vi "Apply Display State to Front Panel and Signal Configuration.vi"(7 "Data In":T1, 10 "references":T2, 11 "Display State In":T3) -> (3 "Display State Out":T3, 5 "Data Out":T1)   [LabVIEW 2017, in "Test Signal Configuration.xctl"]
uses:
  <vilib>/addons/_XControls/Function Generator Configuration/Test Signal Configuration.xctl
  <vilib>/addons/_XControls/Function Generator Configuration/Controls/State.ctl
  <vilib>/addons/_XControls/Function Generator Configuration/Controls/references.ctl
  <vilib>/addons/_XControls/Function Generator Configuration/Controls/Data.ctl
  <vilib>/addons/_NISVFA/_Generation/Signal Generation/SV Signal/SV Signal.lvclass
  <vilib>/addons/_NISVFA/_Generation/Signal Generation/SV Signal/sv_System Timing Model.ctl
  <vilib>/addons/_NISVFA/_Generation/Signal Generation/SV Sinusoid/SV Sinusoid.lvclass
  C:/Program Files (x86)/National Instruments/LabVIEW 2017/vi.lib/addons/_NISVFA/_Generation/Signal Generation/SV Signal/SV Signal.lvclass
  <vilib>/addons/_NISVFA/_Generation/Signal Generation/SV Multitone/SV Multitone.lvclass
  <vilib>/addons/_NISVFA/_Generation/Signal Generation/SV Discrete Sweep/SV Discrete Sweep.lvclass
  C:/Program Files (x86)/National Instruments/LabVIEW 2017/vi.lib/addons/_NISVFA/_Generation/Signal Generation/SV Function/SV Function.lvclass
  <vilib>/addons/_NISVFA/_Generation/Signal Generation/SV Continuous Sweep/SV Continuous Sweep.lvclass
  <vilib>/addons/_NISVFA/_Generation/Signal Generation/SV Noise/SV Noise.lvclass
  <vilib>/addons/_NISVFA/_Generation/Signal Generation/SV Signal/Write Sample Rate.vi
  <vilib>/addons/_NISVFA/_Generation/Signal Generation/SV Signal/Write Minimum Value.vi
  <vilib>/addons/_NISVFA/_Generation/Signal Generation/SV Signal/Write Maximum Value.vi
  <vilib>/addons/_NISVFA/_Generation/Signal Generation/SV Signal/Write DC Offset.vi
  <vilib>/addons/_NISVFA/_Generation/Signal Generation/SV Signal/Write System Timing Model.vi
  <vilib>/addons/_NISVFA/_Generation/Signal Generation/SV Noise/Configure Pink Noise.vi
  <vilib>/addons/_NISVFA/_Generation/Signal Generation/SV Noise/Configure White Noise.vi
  <vilib>/addons/_NISVFA/_Generation/Signal Generation/SV Continuous Sweep/Configure Continuous Sweep.vi
  <vilib>/addons/_NISVFA/_Generation/Signal Generation/SV Signal/Write Measurement Duration.vi
  <vilib>/addons/_NISVFA/_Generation/Signal Generation/SV Function/Write Measurement Cycles.vi
  <vilib>/addons/_NISVFA/_Generation/Signal Generation/SV Discrete Sweep/Configure Frequency Sweep at Constant Amplitude.vi
  <vilib>/addons/_NISVFA/_Generation/Signal Generation/SV Multitone/Configure Multitone (Custom).vi
  <vilib>/addons/_NISVFA/_Generation/Signal Generation/SV Sinusoid/Configure Sine.vi
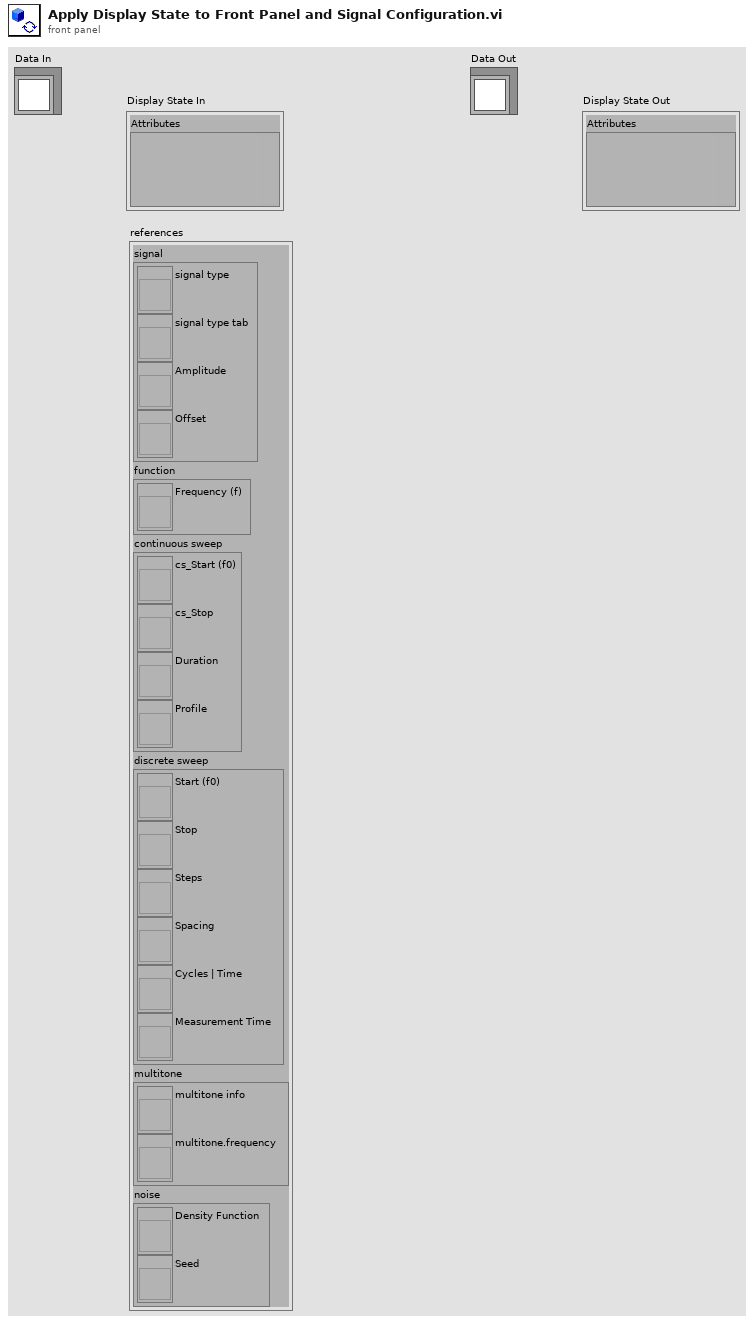
[diagram p1: front panel]
types:
  T1 = typedef "Test Signal Configuration.xctl/Data.ctl" = refnum<class "SV Signal.lvclass">
  T2 = typedef "Test Signal Configuration.xctl/references.ctl" = cluster{"signal":cluster{"signal type":refnum<vi>, "signal type tab":refnum<vi>, "Amplitude":refnum<vi>, "Offset":refnum<vi>}, "function":cluster{"Frequency (f)":refnum<vi>}, "continuous sweep":cluster{"cs_Start (f0)":refnum<vi>, "cs_Stop":refnum<vi>, "Duration":refnum<vi>, "Profile":refnum<vi>}, "discrete sweep":cluster{"Start (f0)":refnum<vi>, "Stop":refnum<vi>, "Steps":refnum<vi>, "Spacing":refnum<vi>, "Cycles | Time":refnum<vi>, "Measurement Time":refnum<vi>}, "multitone":cluster{"multitone info":refnum<vi>, "multitone.frequency":refnum<vi>}, "noise":cluster{"Density Function":refnum<vi>, "Seed":refnum<vi>}}
  T3 = typedef "Test Signal Configuration.xctl/State.ctl" = cluster{"Attributes":variant}
  T4 = typedef "SV Signal.lvclass/sv_System Timing Model.ctl" = i64
  T5 = typedef "Test Signal Configuration.xctl/signal type.ctl" = enum32{"None", "Tone", "Multitone", "Discrete Sweep", "Continuous Sweep", "Noise"}
  T6 = cluster{"Signal":cluster{"Sample Rate":cluster{"name":string, "default":dbl}, "Signal Type":cluster{"name":string, "signal type":T5}, "Amplitude":cluster{"name":string, "default":dbl}, "Offset":cluster{"name":string, "default":dbl}}, "Function":cluster{"Info":cluster{"name":string, "default":variant}, "Type":cluster{"name":string, "default":u16}, "Frequency":cluster{"name":string, "default":dbl}, "Phase":cluster{"name":string, "default":dbl}}, "Continuous Sweep":cluster{"Info":cluster{"name":string, "default":variant}, "Start":cluster{"name":string, "default":dbl}, "Stop":cluster{"name":string, "default":dbl}, "Duration":cluster{"name":string, "default":dbl}, "Profile":cluster{"name":string, "default":enum16{"Linear", "Logarithmic"}}}, "Discrete Sweep":cluster{"Info":cluster{"name":string, "default":variant}, "Start":cluster{"name":string, "default":dbl}, "Stop":cluster{"name":string, "default":dbl}, "Cycles":cluster{"name":string, "default":dbl}, "Time":cluster{"name":string, "default":dbl}, "Spacing":cluster{"name":string, "default":enum16{"Linear", "Logarithmic"}}, "Steps":cluster{"name":string, "default":i32}}, "Multitone":cluster{"Info":cluster{"name":string, "multitone info":cluster{"frequency":dbl, "amplitude":dbl, "phase":dbl}[]}}, "Noise":cluster{"Info":cluster{"name":string, "default":variant}, "Type":cluster{"name":string, "default":u16}, "Amplitude PDF":cluster{"name":string, "default":enum16{"Gaussian", "Rectangular", "Triangular"}}, "Level":cluster{"name":string, "default":dbl}, "Seed":cluster{"name":string, "default":i32}}, "Configuration":cluster{"Min Frequency":cluster{"name":string, "default":dbl}, "Max Frequency":cluster{"name":string, "default":dbl}, "Max Amplitude":cluster{"name":string, "default":dbl}}}
  T7 = enum8{"Enabled", "Disabled", "Disabled and Grayed Out"}
  T8 = cluster{"frequency":dbl, "amplitude":dbl, "phase":dbl}[]
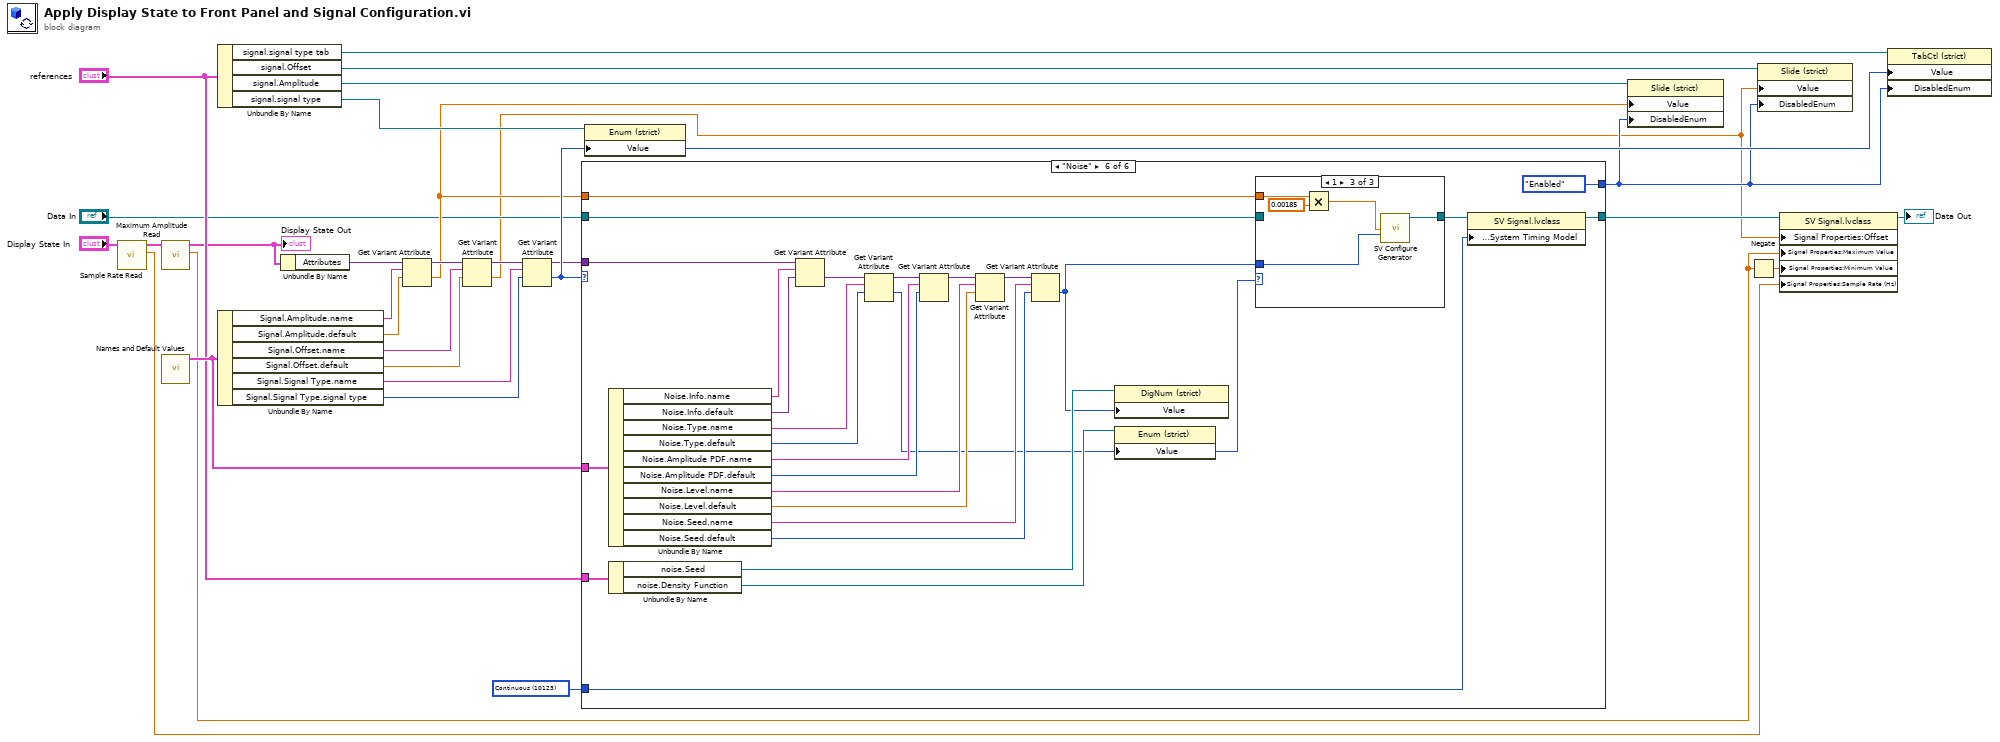
[diagram p0: block diagram]
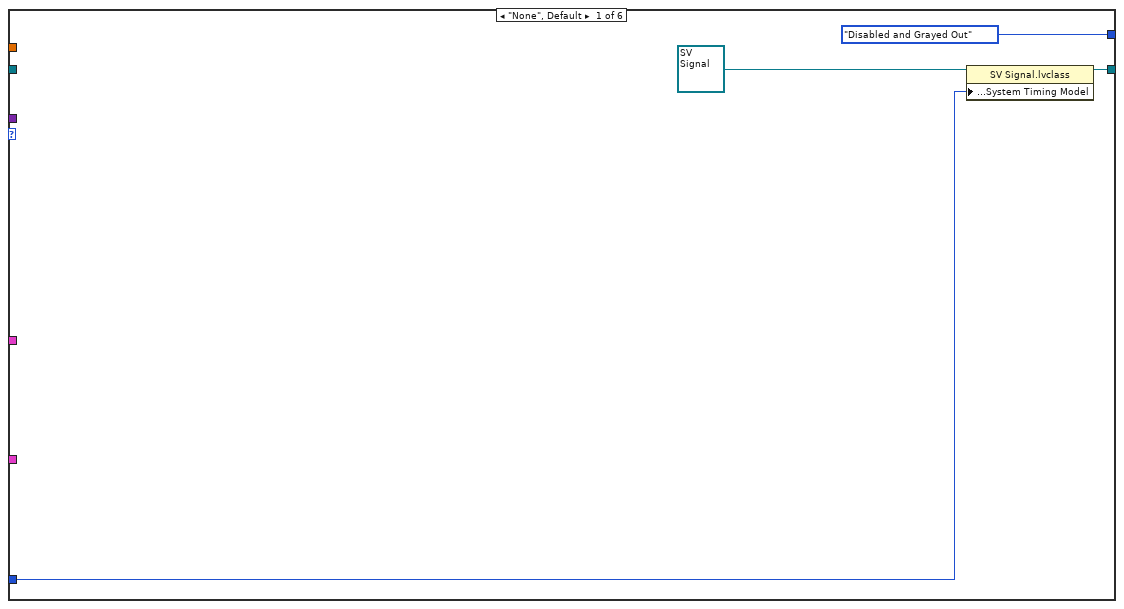
[diagram p2: hidden frame]
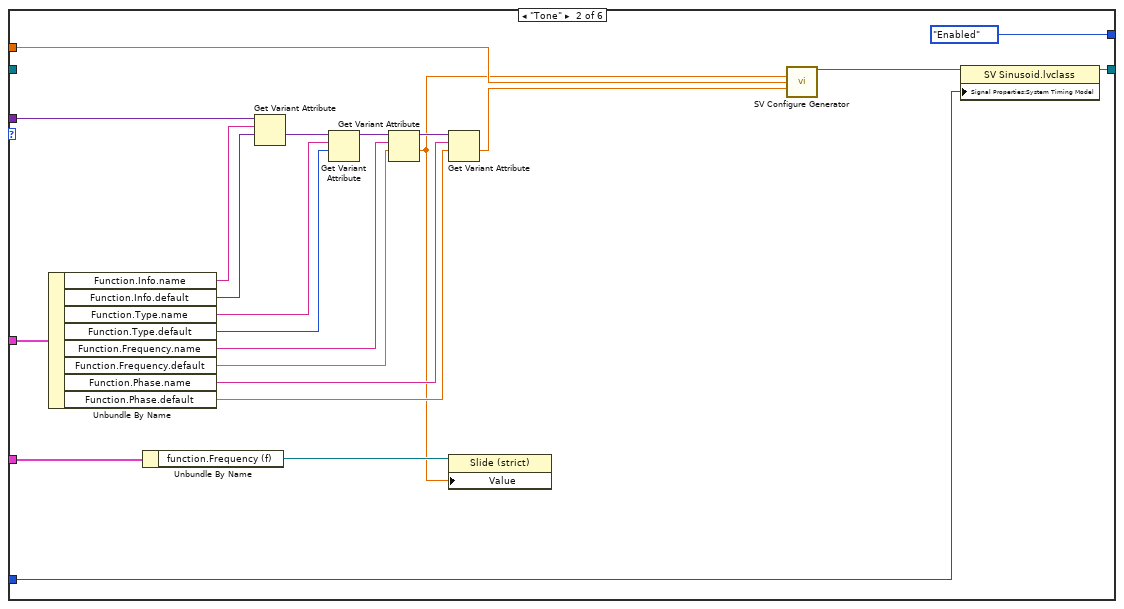
[diagram p3: hidden frame]
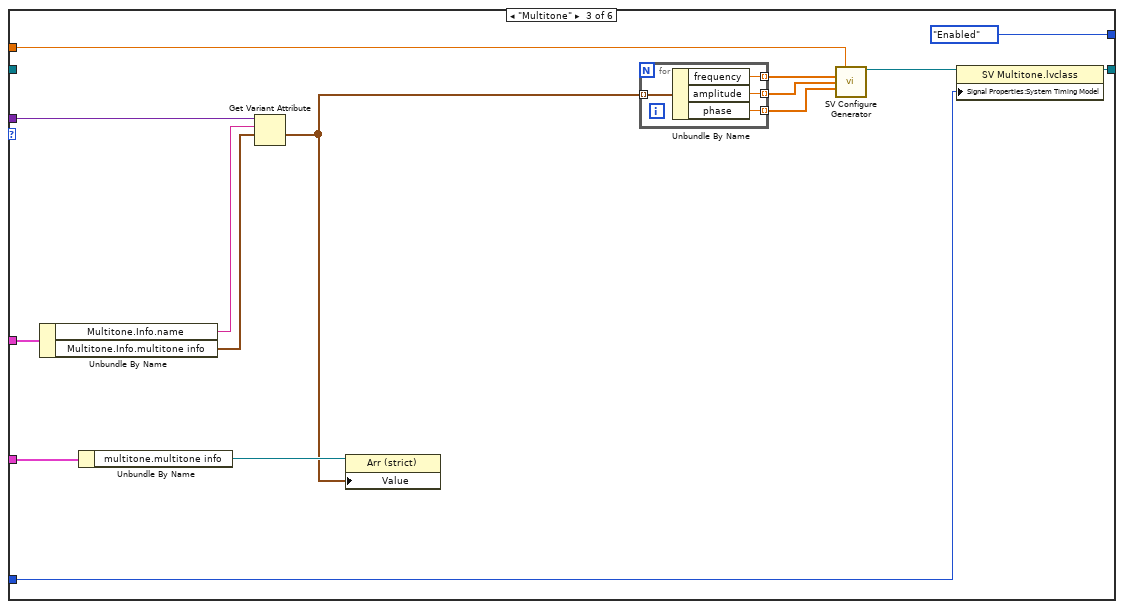
[diagram p4: hidden frame]
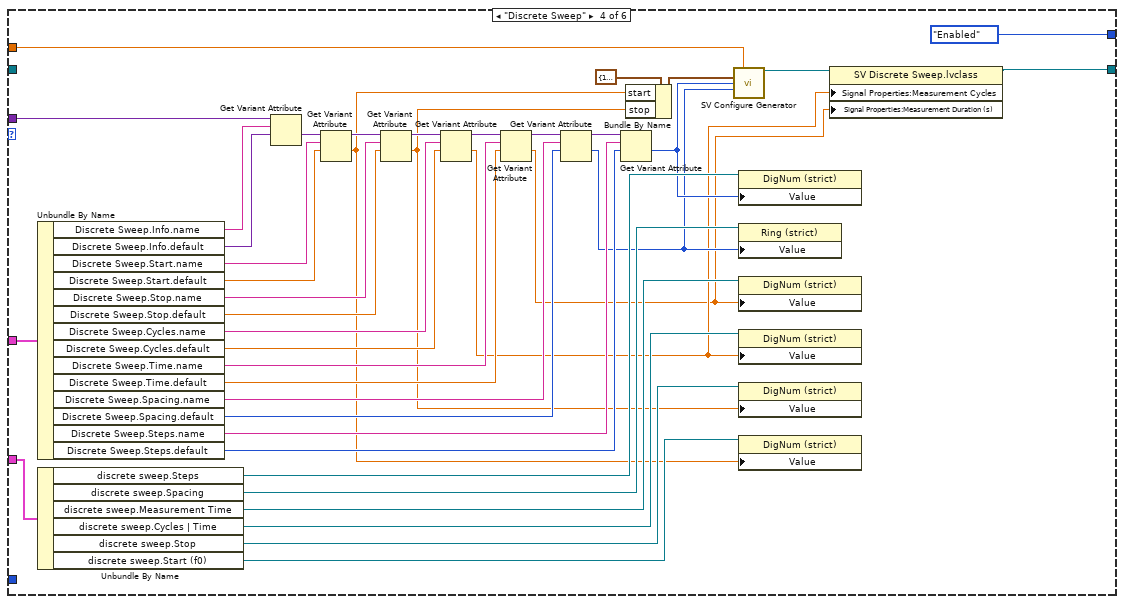
[diagram p5: hidden frame]
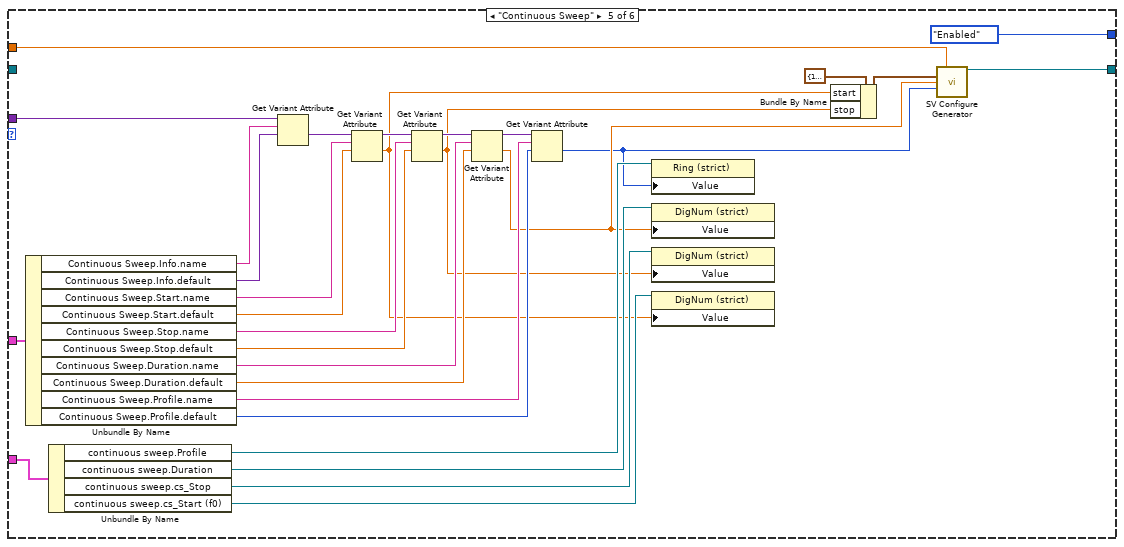
[diagram p6: hidden frame]
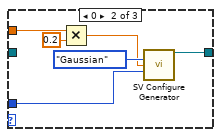
[diagram p8: hidden frame]
diagram:
  w8 = T4 10123 items=["Finite"=10178, "-"=-1, "Continuous"=10123, "-"=-2, "Settled"=110123, "Averaged"=210123, "Discrete Sweep"=310123, "Continuous Sweep"=410123] ("System Timing Model")
  n1 = call <vilib>:"Sample Rate Read.vi"("Display State In"="Display State In") -> ("Value"=w4:dbl, "Display State Out"=w5:T3)  [unwired: 4 in, 1 out]
  n2 = call <vilib>:"Maximum Amplitude Read.vi"("Display State In"=w5) -> ("Value"=w1:dbl, "Display State Out"=w7:T3)  [unwired: 4 in, 1 out]
  "Display State Out" <- w7
  n3 = call <vilib>:"Names and Default Values.vi"() -> ("Names and Default Values"=w14:T6)  [unwired: 11 in]
  n4 = Unbundle By Name("references") -> ("signal.signal type tab"=w25:refnum<vi>, "signal.Offset"=w24:refnum<vi>, "signal.Amplitude"=w23:refnum<vi>, "signal.signal type"=w16:refnum<vi>)
  n5 = Unbundle By Name(w14) -> ("Signal.Amplitude.name"=w30:string, "Signal.Amplitude.default"=w29:dbl, "Signal.Offset.name"=w27:string, "Signal.Offset.default"=w26:dbl, "Signal.Signal Type.name"=w20:string, "Signal.Signal Type.signal type"=w19:T5)
  n6 = Unbundle By Name(w7) -> ("Attributes"=w21:variant)
  n7 = Get Variant Attribute(Variant=w21, name=w30, default value (empty Variant)=w29) -> (duplicate Variant=w28:variant, value=w12:dbl)  [unwired: 1 in, 2 out]
  n8 = Get Variant Attribute(Variant=w28, name=w27, default value (empty Variant)=w26) -> (duplicate Variant=w18:variant, value=w3:dbl)  [unwired: 1 in, 2 out]
  n9 = Get Variant Attribute(Variant=w18, name=w20, default value (empty Variant)=w19) -> (duplicate Variant=w17:variant, value=w22:T5)  [unwired: 1 in, 2 out]
  n10 = case shown="\"Noise\"" w22 {
    tunnel: w17 -> [_ w54 w70 w113 w141 w168]
    tunnel: [T7."Disabled and Grayed Out" ("Disabled") T7."Enabled" ("Disabled") T7."Enabled" ("Disabled") T7."Enabled" ("Disabled") T7."Enabled" ("Disabled") T7."Enabled" ("Disabled")] -> w15
    tunnel: w14 -> [_ w55 w69 w112 w146 w173]
    tunnel: "references" -> [_ w42 w66 w93 w129 w156]
    tunnel: w12 -> [_ w40 w61 w82 w121 w151]
    tunnel: "Data In" -> [_ _ _ _ _ w150]
    tunnel: [w32 w36 w58 w83 w122 w148] -> w10
    tunnel: w8 -> [w31 w35 w57 _ _ w147]
    frame "None", Default {
      n11 = property class="SV Signal.lvclass"(reference=T1 refnum ("Data In"), "Signal Properties:System Timing Model"=w31) -> (reference out=w32:T1)  [unwired: 1 in, 1 out]
    }
    frame "Tone" {
      n12 = Unbundle By Name(w55) -> ("Function.Info.name"=w53:string, "Function.Info.default"=w52:variant, "Function.Type.name"=w50:string, "Function.Type.default"=w49:u16, "Function.Frequency.name"=w47:string, "Function.Frequency.default"=w46:dbl, "Function.Phase.name"=w44:string, "Function.Phase.default"=w43:dbl)
      n13 = Unbundle By Name(w42) -> ("function.Frequency (f)"=w41:refnum<vi>)
      n14 = Get Variant Attribute(Variant=w54, name=w53, default value (empty Variant)=w52) -> (value=w51:variant)  [unwired: 1 in, 3 out]
      n15 = Get Variant Attribute(Variant=w51, name=w50, default value (empty Variant)=w49) -> (duplicate Variant=w48:variant)  [unwired: 1 in, 3 out]
      n16 = Get Variant Attribute(Variant=w48, name=w47, default value (empty Variant)=w46) -> (duplicate Variant=w45:variant, value=w39:dbl)  [unwired: 1 in, 2 out]
      n17 = Get Variant Attribute(Variant=w45, name=w44, default value (empty Variant)=w43) -> (value=w38:dbl)  [unwired: 1 in, 3 out]
      n18 = property class="Slide (strict)"(reference=w41, "Value"=w39) -> ()  [unwired: 1 in, 2 out]
      n19 = call-poly <vilib>:"SV Configure Generator.vi"("frequency (Hz)"=w39, "amplitude"=w40, "phase (deg)"=w38) -> ("signal configuration"=w37:refnum<class "SV Sinusoid.lvclass">)  [unwired: 11 in, 1 out]
      n20 = property class="SV Sinusoid.lvclass"(reference=w37, "Signal Properties:System Timing Model"=w35) -> (reference out=w36:refnum<class "SV Sinusoid.lvclass">)  [unwired: 1 in, 1 out]
    }
    frame "Multitone" {
      n21 = Unbundle By Name(w69) -> ("Multitone.Info.name"=w68:string, "Multitone.Info.multitone info"=w67:T8)
      n22 = Unbundle By Name(w66) -> ("multitone.multitone info"=w65:refnum<vi>)
      n23 = Get Variant Attribute(Variant=w70, name=w68, default value (empty Variant)=w67) -> (value=w60:T8)  [unwired: 1 in, 3 out]
      n24 = property class="Arr (strict)"(reference=w65, "Value"=w60) -> ()  [unwired: 1 in, 2 out]
      n25 = for {
        tunnel: w60 -> [w75] mode=indexing
        tunnel: [w74] -> w64 mode=indexing
        tunnel: [w73] -> w63 mode=indexing
        tunnel: [w72] -> w62 mode=indexing
        n26 = Unbundle By Name(w75) -> ("frequency"=w74:dbl, "amplitude"=w73:dbl, "phase"=w72:dbl)
      }
      n27 = call-poly <vilib>:"SV Configure Generator.vi"("overall amplitude"=w61, "frequencies [Hz]"=w64, "amplitudes"=w63, "phases [deg]"=w62) -> ("signal configuration"=w59:refnum<class "SV Multitone.lvclass">)  [unwired: 9 in, 2 out]
      n28 = property class="SV Multitone.lvclass"(reference=w59, "Signal Properties:System Timing Model"=w57) -> (reference out=w58:refnum<class "SV Multitone.lvclass">)  [unwired: 1 in, 1 out]
    }
    frame "Discrete Sweep" {
      n29 = Unbundle By Name(w112) -> ("Discrete Sweep.Info.name"=w111:string, "Discrete Sweep.Info.default"=w110:variant, "Discrete Sweep.Start.name"=w109:string, "Discrete Sweep.Start.default"=w108:dbl, "Discrete Sweep.Stop.name"=w107:string, "Discrete Sweep.Stop.default"=w106:dbl, "Discrete Sweep.Cycles.name"=w105:string, "Discrete Sweep.Cycles.default"=w104:dbl, "Discrete Sweep.Time.name"=w100:string, "Discrete Sweep.Time.default"=w99:dbl, "Discrete Sweep.Spacing.name"=w98:string, "Discrete Sweep.Spacing.default"=w97:enum16{"Linear", "Logarithmic"}, "Discrete Sweep.Steps.name"=w96:string, "Discrete Sweep.Steps.default"=w95:i32)
      n30 = Unbundle By Name(w93) -> ("discrete sweep.Steps"=w87:refnum<vi>, "discrete sweep.Spacing"=w88:refnum<vi>, "discrete sweep.Measurement Time"=w89:refnum<vi>, "discrete sweep.Cycles | Time"=w90:refnum<vi>, "discrete sweep.Stop"=w91:refnum<vi>, "discrete sweep.Start (f0)"=w92:refnum<vi>)
      n31 = Get Variant Attribute(Variant=w113, name=w111, default value (empty Variant)=w110) -> (value=w116:variant)  [unwired: 1 in, 3 out]
      n32 = Get Variant Attribute(Variant=w116, name=w109, default value (empty Variant)=w108) -> (duplicate Variant=w115:variant, value=w81:dbl)  [unwired: 1 in, 2 out]
      n33 = Get Variant Attribute(Variant=w115, name=w107, default value (empty Variant)=w106) -> (duplicate Variant=w114:variant, value=w80:dbl)  [unwired: 1 in, 2 out]
      n34 = Get Variant Attribute(Variant=w114, name=w105, default value (empty Variant)=w104) -> (duplicate Variant=w101:variant, value=w77:dbl)  [unwired: 1 in, 2 out]
      n35 = Get Variant Attribute(Variant=w101, name=w100, default value (empty Variant)=w99) -> (duplicate Variant=w102:variant, value=w76:dbl)  [unwired: 1 in, 2 out]
      n36 = Get Variant Attribute(Variant=w102, name=w98, default value (empty Variant)=w97) -> (duplicate Variant=w103:variant, value=w78:enum16{"Linear", "Logarithmic"})  [unwired: 1 in, 2 out]
      n37 = Get Variant Attribute(Variant=w103, name=w96, default value (empty Variant)=w95) -> (value=w79:i32)  [unwired: 1 in, 3 out]
      n38 = Bundle By Name(cluster=cluster{"start":dbl, "stop":dbl} {"start"=10.0, "stop"=10000.0} ("frequency range [Hz]"), "start"=w81, "stop"=w80) -> (w84:cluster{"start":dbl, "stop":dbl})
      n39 = call-poly <vilib>:"SV Configure Generator.vi"("amplitude"=w82, "frequency range [Hz]"=w84, "number of steps"=w79, "profile"=w78) -> ("signal configuration"=w85:refnum<class "SV Discrete Sweep.lvclass">)  [unwired: 10 in, 1 out]
      n40 = property class="DigNum (strict)"(reference=w87, "Value"=w79) -> ()  [unwired: 1 in, 2 out]
      n41 = property class="Ring (strict)"(reference=w88, "Value"=w78) -> ()  [unwired: 1 in, 2 out]
      n42 = property class="DigNum (strict)"(reference=w89, "Value"=w76) -> ()  [unwired: 1 in, 2 out]
      n43 = property class="DigNum (strict)"(reference=w90, "Value"=w77) -> ()  [unwired: 1 in, 2 out]
      n44 = property class="DigNum (strict)"(reference=w91, "Value"=w80) -> ()  [unwired: 1 in, 2 out]
      n45 = property class="DigNum (strict)"(reference=w92, "Value"=w81) -> ()  [unwired: 1 in, 2 out]
      n46 = property class="SV Discrete Sweep.lvclass"(reference=w85, "Signal Properties:Measurement Cycles"=w77, "Signal Properties:Measurement Duration (s)"=w76) -> (reference out=w83:refnum<class "SV Discrete Sweep.lvclass">)  [unwired: 1 in, 1 out]
    }
    frame "Continuous Sweep" {
      n47 = Unbundle By Name(w146) -> ("Continuous Sweep.Info.name"=w140:string, "Continuous Sweep.Info.default"=w139:variant, "Continuous Sweep.Start.name"=w138:string, "Continuous Sweep.Start.default"=w137:dbl, "Continuous Sweep.Stop.name"=w136:string, "Continuous Sweep.Stop.default"=w135:dbl, "Continuous Sweep.Duration.name"=w134:string, "Continuous Sweep.Duration.default"=w133:dbl, "Continuous Sweep.Profile.name"=w132:string, "Continuous Sweep.Profile.default"=w131:enum16{"Linear", "Logarithmic"})
      n48 = Unbundle By Name(w129) -> ("continuous sweep.Profile"=w125:refnum<vi>, "continuous sweep.Duration"=w126:refnum<vi>, "continuous sweep.cs_Stop"=w127:refnum<vi>, "continuous sweep.cs_Start (f0)"=w128:refnum<vi>)
      n49 = Get Variant Attribute(Variant=w141, name=w140, default value (empty Variant)=w139) -> (value=w145:variant)  [unwired: 1 in, 3 out]
      n50 = Get Variant Attribute(Variant=w145, name=w138, default value (empty Variant)=w137) -> (duplicate Variant=w144:variant, value=w120:dbl)  [unwired: 1 in, 2 out]
      n51 = Get Variant Attribute(Variant=w144, name=w136, default value (empty Variant)=w135) -> (duplicate Variant=w143:variant, value=w119:dbl)  [unwired: 1 in, 2 out]
      n52 = Get Variant Attribute(Variant=w143, name=w134, default value (empty Variant)=w133) -> (duplicate Variant=w142:variant, value=w118:dbl)  [unwired: 1 in, 2 out]
      n53 = Get Variant Attribute(Variant=w142, name=w132, default value (empty Variant)=w131) -> (value=w117:enum16{"Linear", "Logarithmic"})  [unwired: 1 in, 3 out]
      n54 = property class="Ring (strict)"(reference=w125, "Value"=w117) -> ()  [unwired: 1 in, 2 out]
      n55 = property class="DigNum (strict)"(reference=w126, "Value"=w118) -> ()  [unwired: 1 in, 2 out]
      n56 = property class="DigNum (strict)"(reference=w127, "Value"=w119) -> ()  [unwired: 1 in, 2 out]
      n57 = property class="DigNum (strict)"(reference=w128, "Value"=w120) -> ()  [unwired: 1 in, 2 out]
      n58 = Bundle By Name(cluster=cluster{"start":dbl, "stop":dbl} {"start"=10.0, "stop"=10000.0} ("frequency range [Hz]"), "start"=w120, "stop"=w119) -> (w123:cluster{"start":dbl, "stop":dbl})
      n59 = call-poly <vilib>:"SV Configure Generator.vi"("amplitude"=w121, "frequency range [Hz]"=w123, "duration [s]"=w118, "profile"=w117) -> ("signal configuration"=w122:refnum<class "SV Continuous Sweep.lvclass">)  [unwired: 10 in, 1 out]
    }
    frame "Noise" {
      n60 = Unbundle By Name(w173) -> ("Noise.Info.name"=w167:string, "Noise.Info.default"=w166:variant, "Noise.Type.name"=w165:string, "Noise.Type.default"=w164:u16, "Noise.Amplitude PDF.name"=w163:string, "Noise.Amplitude PDF.default"=w162:enum16{"Gaussian", "Rectangular", "Triangular"}, "Noise.Level.name"=w161:string, "Noise.Level.default"=w160:dbl, "Noise.Seed.name"=w159:string, "Noise.Seed.default"=w158:i32)
      n61 = Unbundle By Name(w156) -> ("noise.Seed"=w155:refnum<vi>, "noise.Density Function"=w154:refnum<vi>)
      n62 = Get Variant Attribute(Variant=w168, name=w167, default value (empty Variant)=w166) -> (value=w172:variant)  [unwired: 1 in, 3 out]
      n63 = Get Variant Attribute(Variant=w172, name=w165, default value (empty Variant)=w164) -> (duplicate Variant=w171:variant, value=w152:u16)  [unwired: 1 in, 2 out]
      n64 = Get Variant Attribute(Variant=w171, name=w163, default value (empty Variant)=w162) -> (duplicate Variant=w170:variant)  [unwired: 1 in, 3 out]
      n65 = Get Variant Attribute(Variant=w170, name=w161, default value (empty Variant)=w160) -> (duplicate Variant=w169:variant)  [unwired: 1 in, 3 out]
      n66 = Get Variant Attribute(Variant=w169, name=w159, default value (empty Variant)=w158) -> (value=w153:i32)  [unwired: 1 in, 3 out]
      n67 = property class="DigNum (strict)"(reference=w155, "Value"=w153) -> ()  [unwired: 1 in, 2 out]
      n68 = property class="Enum (strict)"(reference=w154, "Value"=w152) -> ()  [unwired: 1 in, 2 out]
      n69 = case shown="1" w152 {
        tunnel: [w174 w180 w185] -> w149
        tunnel: w151 -> [_ w176 w182]
        tunnel: w153 -> [_ w178 w184]
        tunnel: w150 -> [w174 _ _]
        frame Default {
        }
        frame 0 {
          n70 = Multiply(x=w176, y=0.2) -> (x*y=w175:dbl)
          n71 = call-poly <vilib>:"SV Configure Generator.vi"("amplitude PDF"=enum16{"Gaussian", "Rectangular", "Triangular"}."Gaussian", "level"=w175, "seed"=w178) -> ("signal configuration"=w180:refnum<class "SV Noise.lvclass">)  [unwired: 11 in, 1 out]
        }
        frame 1 {
          n72 = Multiply(x=w182, y=0.00185) -> (x*y=w181:dbl)
          n73 = call-poly <vilib>:"SV Configure Generator.vi"("level"=w181, "seed"=w184) -> ("signal configuration"=w185:refnum<class "SV Noise.lvclass">)  [unwired: 12 in, 1 out]
        }
      }
      n74 = property class="SV Signal.lvclass"(reference=w149, "Signal Properties:System Timing Model"=w147) -> (reference out=w148:T1)  [unwired: 1 in, 1 out]
    }
  }
  n75 = property class="Enum (strict)"(reference=w16, "Value"=w22) -> ()  [unwired: 1 in, 2 out]
  n76 = property class="Slide (strict)"(reference=w23, "Value"=w12, "DisabledEnum"=w15) -> ()  [unwired: 1 in, 2 out]
  n77 = Negate(x=w1) -> (-x=w2:dbl)
  n78 = property class="Slide (strict)"(reference=w24, "Value"=w3, "DisabledEnum"=w15) -> ()  [unwired: 1 in, 2 out]
  n79 = property class="SV Signal.lvclass"(reference=w10, "Signal Properties:Offset"=w3, "Signal Properties:Maximum Value"=w1, "Signal Properties:Minimum Value"=w2, "Signal Properties:Sample Rate (Hz)"=w4) -> (reference out=→"Data Out":T1)  [unwired: 1 in, 1 out]
  n80 = property class="TabCtl (strict)"(reference=w25, "Value"=w22, "DisabledEnum"=w15) -> ()  [unwired: 1 in, 2 out]
